vi "Assert Matches Regular Expression.vi"(7 "Label":string="Assert Matches Regular Expression", 8 "error in (no error)":errorcluster, 10 "Actual Value":string, 11 "Regular Expression":string) -> (0 "error out":errorcluster)   [LabVIEW 2017, in "Assert Extensions.lvclass"]
doc: "Assert that <B>actual value</B> matches <B>regular expression</B>."
uses:
  Assert Extensions.lvclass
  <vilib>/addons/_JKI Toolkits/Caraya/classes/Properties.Assert/Properties.Assert.lvclass
  C:/Program Files/National Instruments/LabVIEW 2017/vi.lib/addons/_JKI Toolkits/Caraya/classes/Properties/Properties.lvclass
  <vilib>/regexp/Match Regular Expression.xnode
  <vilib>/addons/_JKI Toolkits/Caraya/classes/Properties/Properties.lvclass
  <vilib>/addons/_JKI Toolkits/Caraya/classes/Assert/Assert.lvclass
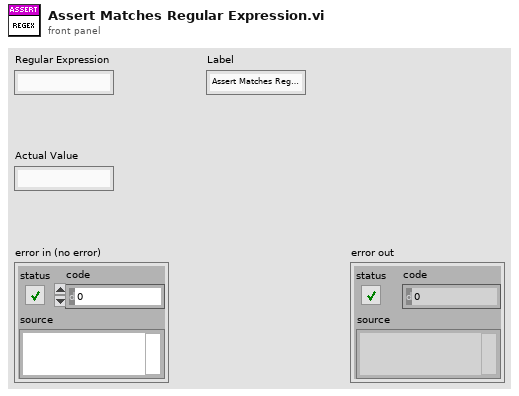
[diagram p1: front panel]
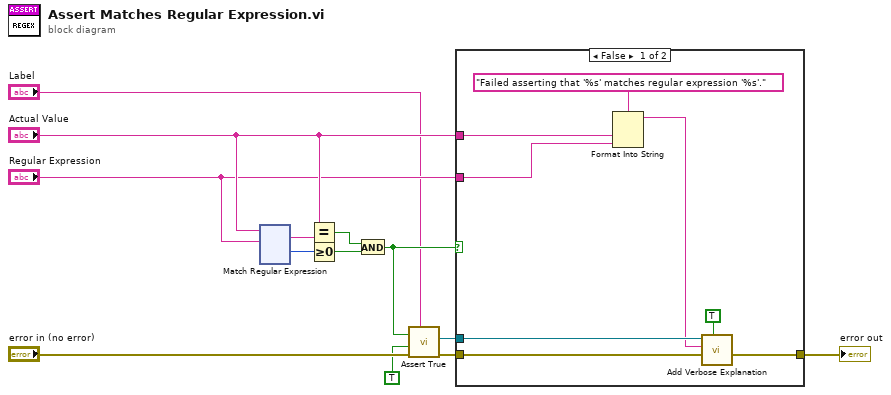
[diagram p0: block diagram]
diagram:
  n1 = xnode "Match Regular Expression"("input string"="Actual Value", "regular expression"="Regular Expression") -> ("whole match"=w9:string, "offset past match"=w6:i32)  [unwired: 4 in, 3 out]
  n2 = Equal?(x="Actual Value", y=w9) -> (x = y?=w7:bool)
  n3 = Greater Or Equal To 0?(x=w6) -> (x >= 0?=w8:bool)
  n4 = And(x=w7, y=w8) -> (x .and. y?=w5:bool)
  n5 = call <vilib>:"Assert True.vi"("Label"="Label", "error in (no error)"="error in (no error)", "Register with caller test (F)"=TRUE, "True?"=w5) -> ("error out"=w12:errorcluster, "Properties"=w10:refnum<class "Properties.Assert.lvclass">)  [unwired: 6 in]
  n6 = case shown="False" w5 {
    tunnel: w12 -> [w21 w22]
    tunnel: [w20 w22] -> w11
    tunnel: w10 -> [w19 _]
    tunnel: "Actual Value" -> [w15 _]
    tunnel: "Regular Expression" -> [w14 _]
    frame False {
      n7 = Format Into String(format string="Failed asserting that '%s' matches regular expression '%s'.", w15, w14) -> (resulting string=w16:string)  [unwired: 2 in, 1 out]
      n8 = call <vilib>:"Add Verbose Explanation.vi"("overwrite?"=TRUE, "error in (no error)"=w21, "Verbose Explanation"=w16, "Properties"=w19) -> ("error out"=w20:errorcluster)  [unwired: 6 in, 1 out]
    }
    frame True {
    }
  }
  "error out" <- w11
